vi "Close Host Stream Command Queue.vi"(8 "error in (no error)":errorcluster, 11 "Cmd Q":refnum<queue>) -> (0 "error out":errorcluster)   [LabVIEW 2019, in "CAN Stream Support Workspace Shared.lvlib"]
uses:
  CAN Stream Support Workspace Shared.lvlib
  Types/Host Stream Queue Type.ctl
  Types/Host Stream Queue Command.ctl
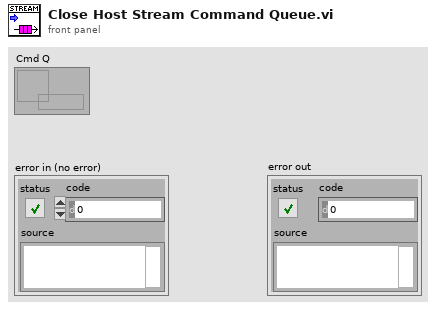
[diagram p1: front panel]
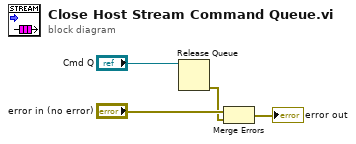
[diagram p0: block diagram]
diagram:
  n1 = Release Queue(queue="Cmd Q") -> (error out=w2:errorcluster)  [unwired: 2 in, 2 out]
  n2 = Merge Errors("error in (no error)", w2) -> (→"error out":errorcluster)
